vi "tslin_set_node_funtiontype.vi"(8 "错误输入（无错误）":errorcluster, 9 "set_node_funtiontype":i32(ring) items=["MasterNode", "SlaveNode", "MonitorNote"], 10 "AAppChannel":i32(ring) items=["CHN1", "CHN2", "CHN3", "CHN4", "CHN5", "CHN6", "CHN7", "CHN8", "CHN9", "CHN10", "CHN11", "CHN12", "CHN13", "CHN14", "CHN15", "CHN16", "CHN17", "CHN18", "CHN19", "CHN20", "CHN21", "CHN22", "CHN23", "CHN24", "CHN25", "CHN26", "CHN27", "CHN28", "CHN29", "CHN30", "CHN31", "CHN32"], 11 "path":path) -> (0 "错误输出":errorcluster, 2 "return":i32, 3 "path out":path)   [LabVIEW 2014]
doc: "Function Introduction :\nSet the working mode of the specified channel (master, slave, listening mode)\nCall location :\ninput parameter :\nAIdxChn: Channel Index\nAFunctionType: lin node type\n0：T_MasterNode 1：T_SlaveNode 2: T_MonitorNode\nReturn value :\n0: Execution successful\nOther values: Failed"
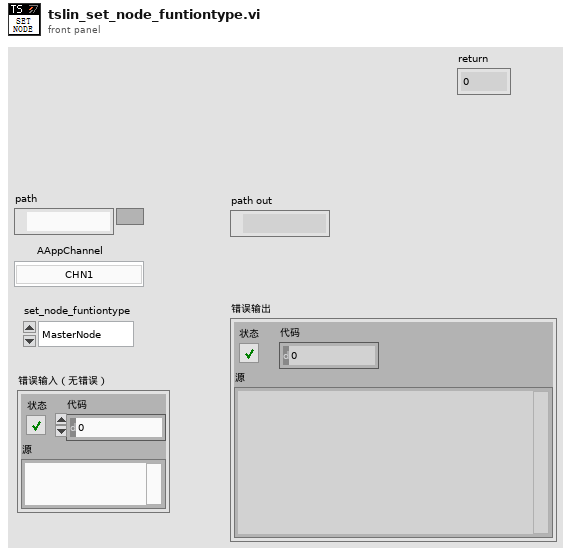
[diagram p1: front panel]
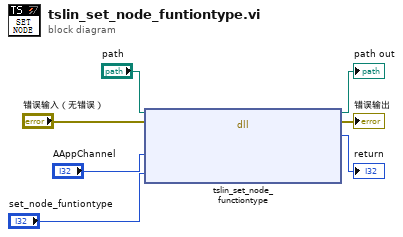
[diagram p0: block diagram]
diagram:
  n1 = dll-call lib="D:/Program Files (x86)/TOSUN/TSMaster/Data/SDK/lib/x86/TSMaster.dll" fn="tslin_set_node_functiontype"(path in="path", error in="错误输入（无错误）", "AChnIdx"="AAppChannel", "AFunctionType"="set_node_funtiontype") -> (path out=→"path out":path, error out=→"错误输出":errorcluster, "tslin_set_node_funtiontype"=→"return":i32)  [unwired: 3 in]
